vi "Sum of Partial Sums.vi"(8 "delta_x":dbl format="%_6g", 9 "Number of Partial Sum":i32, 11 "Array":dbl[](array[numeric]) format="%_6g") -> (2 "Simp Value":dbl)   [LabVIEW 2017]
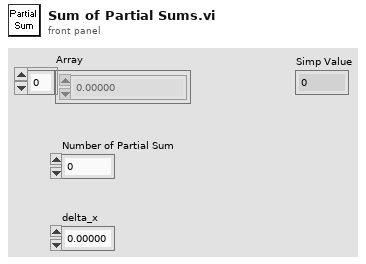
[diagram p1: front panel]
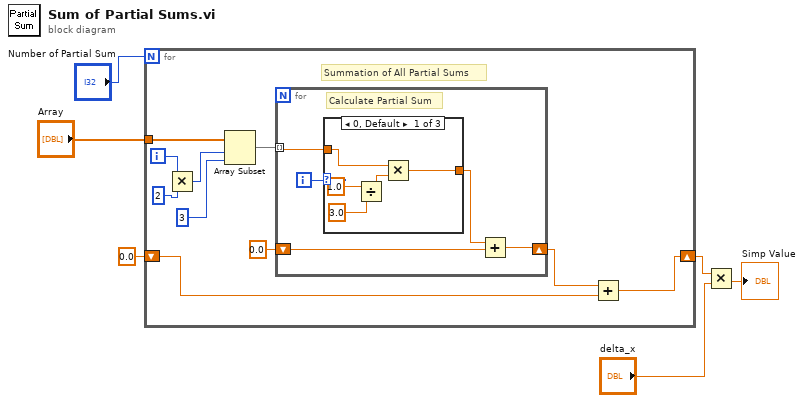
[diagram p0: block diagram]
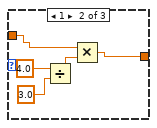
[diagram p2: hidden frame]
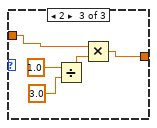
[diagram p3: hidden frame]
diagram:
  n1 = for {
    N: "Number of Partial Sum" -> [_]
    tunnel: "Array" -> [w16]
    shift-right: [w7] -> w2
    shift-left: 0.0 -> [w8]
    i -> [w11]
    # "Summation of All Partial Sums"
    n2 = Multiply(x=w11, y=2 ("length")) -> (x*y=w10:i32)
    n3 = Array Subset(array=w16, index=w10, length=3) -> (w14:dbl[])
    n4 = for {
      tunnel: w14 -> [w20] mode=indexing
      shift-right: [w18] -> w9
      shift-left: 0.0 -> [w17]
      i -> [w21]
      # "Calculate Partial Sum"
      n5 = case shown="0, Default" w21 {
        tunnel: w20 -> [w23 w28 w33]
        tunnel: [w22 w27 w32] -> w19
        frame 0, Default {
          n6 = Divide(x=1.0, y=3.0) -> (x/y=w24:dbl)
          n7 = Multiply(x=w23, y=w24) -> (x*y=w22:dbl)
        }
        frame 1 {
          n8 = Divide(x=4.0, y=3.0) -> (x/y=w31:dbl)
          n9 = Multiply(x=w28, y=w31) -> (x*y=w27:dbl)
        }
        frame 2 {
          n10 = Divide(x=1.0, y=3.0) -> (x/y=w36:dbl)
          n11 = Multiply(x=w33, y=w36) -> (x*y=w32:dbl)
        }
      }
      n12 = Add(x=w19, y=w17) -> (x+y=w18:dbl)
    }
    n13 = Add(x=w9, y=w8) -> (x+y=w7:dbl)
  }
  n14 = Multiply(x=w2, y="delta_x") -> (x*y=→"Simp Value":dbl)
